vi "SeCrTs-Drive_Read_L.vi"(8 "error in":errorcluster, 9 "Message Queue":refnum<queue>, 11 "Data FIFO Ref":T1) -> (0 "error out":errorcluster)   [LabVIEW 2022 SP3]
uses:
  RT Controls/SeCrTs-Data FIFO.ctl
  RT Support/SeCrTs-RT_Global_R.vi
panel:
  in  "TCP_Port_Bottom":u16=3000
  in  "TCP_Port_Top":u16=2000
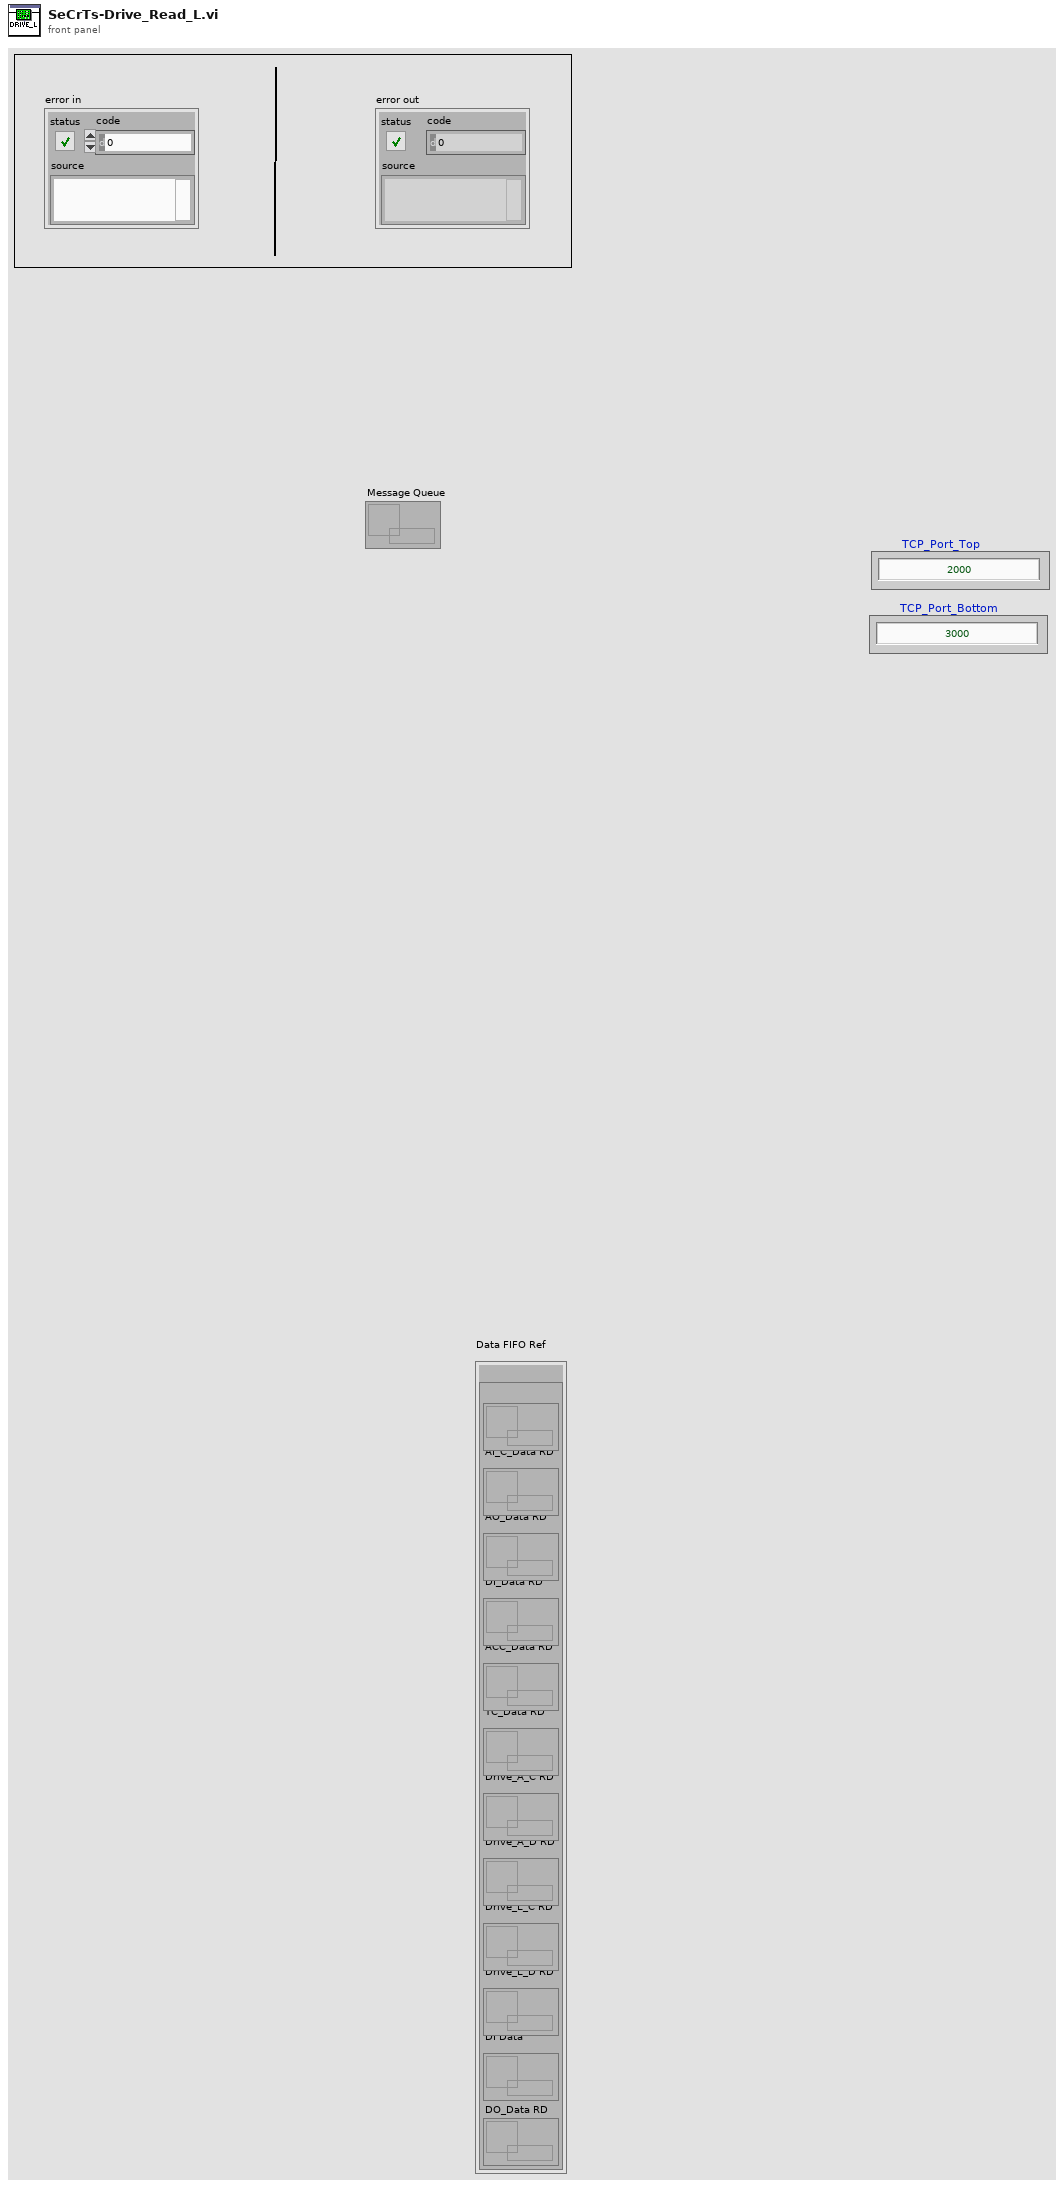
[diagram p1: front panel]
types:
  T1 = typedef "SeCrTs-Data FIFO.ctl" = cluster{"RD":cluster{"AI_V_Data RD":refnum<queue>, "AI_C_Data RD":refnum<queue>, "AO_Data RD":refnum<queue>, "DI_Data RD":refnum<queue>, "ACC_Data RD":refnum<queue>, "TC_Data RD":refnum<queue>, "Drive_A_C RD":refnum<queue>, "Drive_A_D RD":refnum<queue>, "Drive_L_C RD":refnum<queue>, "Drive_L_D RD":refnum<queue>, "DI Data":refnum<queue>, "DO_Data RD":refnum<queue>}}
  T2 = enum16{"AI C", "AI V", "AO", "DI", "DO", "TC", "ACC", "DR L", "DR A"}
  T3 = enum16{"Init", "Read 'All'", "Read 'n'", "Read '1'", "Write '1'", "Write 'n'", "Write 'All'"}
  T4 = cluster{"Start DAQ":bool, "Stop DAQ":bool, "RT Stop":bool, "RT Exit":bool, "Start Seq":bool}
  T5 = cluster{"En_Drive_A":bool, "En_Drive_L":bool, "Exit_Drive_A":bool, "Exit_Drive_L":bool}
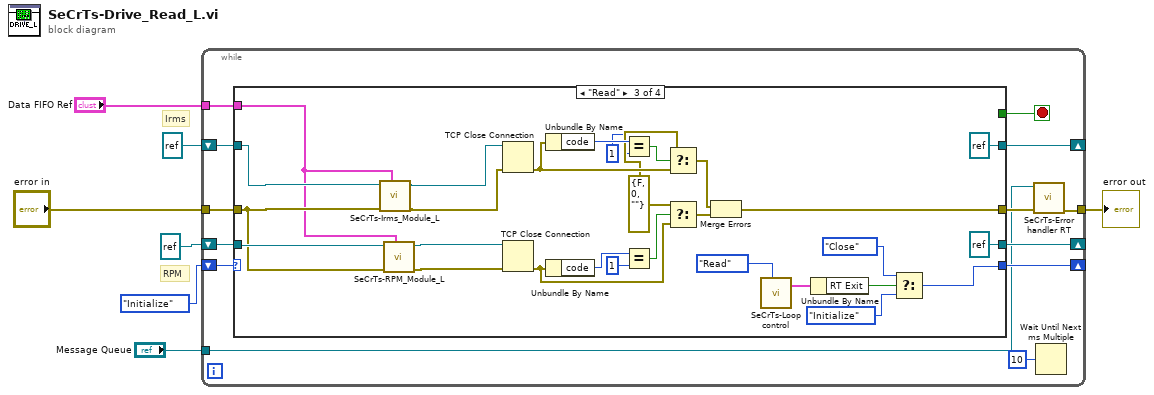
[diagram p0: block diagram]
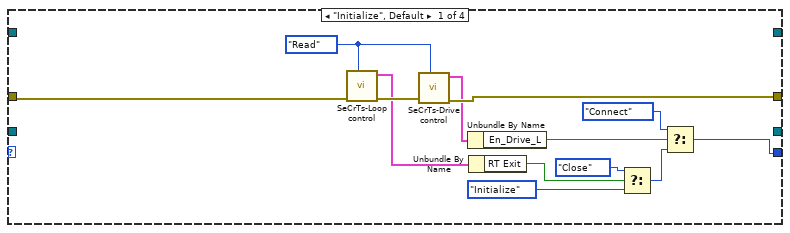
[diagram p2: hidden frame]
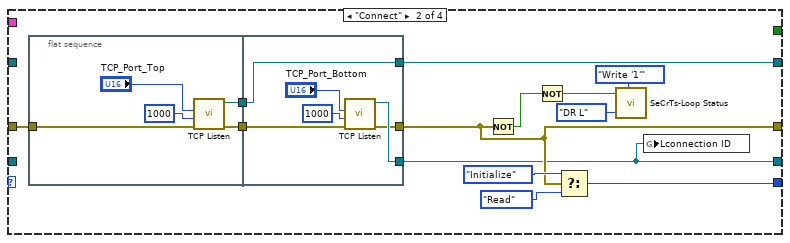
[diagram p3: hidden frame]
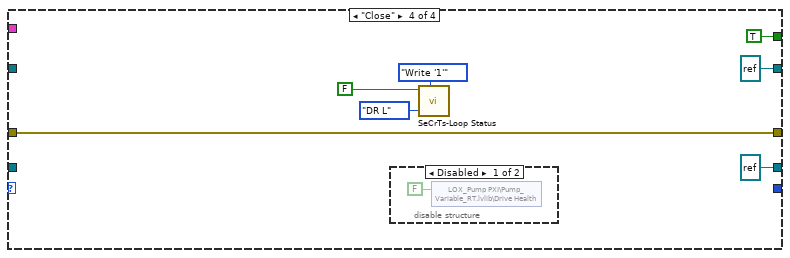
[diagram p4: hidden frame]
diagram:
  # "RPM"
  # "Irms"
  n1 = while {
    shift-right: [w19] -> _
    shift-left: enum16{"Initialize", "Connect", "Read", "Close"}."Initialize" -> [w20]
    tunnel: "error in" -> [w18]
    tunnel: [w10] -> w5
    shift-right: [w17] -> _
    shift-left: refnum<k5> refnum ("connection ID") -> [w15]
    shift-right: [w16] -> _
    shift-left: refnum<k5> refnum ("connection ID") -> [w14]
    tunnel: "Data FIFO Ref" -> [w12]
    tunnel: "Message Queue" -> [w9]
    stop <- w13 stop-if-true
    n2 = case shown="\"Read\"" w20 {
      tunnel: [w33 w40 w83 _] -> w19
      tunnel: w18 -> [w28 w44 w60 w89]
      tunnel: [w26 w39 w71 w89] -> w11
      tunnel: [_ w43 refnum<k5> refnum ("TCP Network Connection out") refnum<k5> refnum ("TCP Network Connection out")] -> w17
      tunnel: [_ w38 refnum<k5> refnum ("TCP Network Connection out") refnum<k5> refnum ("TCP Network Connection out")] -> w16
      tunnel: w15 -> [_ _ w65 _]
      tunnel: w14 -> [_ _ w61 _]
      tunnel: [_ _ _ TRUE] -> w13
      tunnel: w12 -> [_ _ w58 _]
      frame "Initialize", Default {
        w25 = enum16{"Init", "Write", "Read"}."Read" ("Action")
        n3 = call "SeCrTs-Loop control.vi"("Action"=w25, "error in (no error)"=w28) -> ("error Out"=w27:errorcluster, "Loop Control out"=w24:T4)  [unwired: 8 in]
        n4 = call "SeCrTs-Drive control.vi"("Action"=w25, "error in"=w27) -> ("error Out"=w26:errorcluster, "Loop Control Out"=w22:T5)  [unwired: 8 in]
        n5 = Unbundle By Name(w22) -> ("En_Drive_L"=w21:bool)
        n6 = Unbundle By Name(w24) -> ("RT Exit"=w23:bool)
        n7 = Select(t=enum16{"Initialize", "Connect", "Read", "Close"}."Close", s=w23, f=enum16{"Initialize", "Connect", "Read", "Close"}."Initialize") -> (s? t:f=w29:enum16{"Initialize", "Connect", "Read", "Close"})
        n8 = Select(t=enum16{"Initialize", "Connect", "Read", "Close"}."Connect", s=w21, f=w29) -> (s? t:f=w33:enum16{"Initialize", "Connect", "Read", "Close"})
      }
      frame "Connect" {
        n9 = flat-sequence {
          tunnel: w44 -> [w49]
          tunnel: [w48] -> w46
          tunnel: [w47] -> w45
          tunnel: [w57] -> w38
          tunnel: w46 -> [w53]
          tunnel: w45 -> [w56]
          tunnel: [w56] -> w43
          tunnel: [w52] -> w39
          frame #0 {
            n10 = call <vilib>:"TCP Listen.vi"("error in (no error)"=w49, "timeout ms (wait forever: -1)"=1000, "port"="TCP_Port_Top") -> ("error out"=w48:errorcluster, "connection ID"=w47:refnum<k5>)  [unwired: 4 in, 3 out]
          }
          frame #1 {
            n11 = call <vilib>:"TCP Listen.vi"("error in (no error)"=w53, "timeout ms (wait forever: -1)"=1000, "port"="TCP_Port_Bottom") -> ("error out"=w52:errorcluster, "connection ID"=w57:refnum<k5>)  [unwired: 4 in, 3 out]
          }
        }
        n12 = Not(x=w39) -> (.not. x?=w34:bool)
        n13 = Not(x=w34) -> (.not. x?=w36:bool)
        n14 = Select(t=enum16{"Initialize", "Connect", "Read", "Close"}."Initialize", s=w39, f=enum16{"Initialize", "Connect", "Read", "Close"}."Read") -> (s? t:f=w40:enum16{"Initialize", "Connect", "Read", "Close"})
        n15 = call "SeCrTs-Loop Status.vi"("Option"=T3."Write '1'", "Status"=w36, "Loop"=T2."DR L") -> ()  [unwired: 6 in, 3 out]
        n16 = global write "SeCrTs-RT_Global_R.vi" "Lconnection ID"(w38) -> ()
      }
      frame "Read" {
        w74 = errorcluster {"status"=FALSE, "code"=0, "source"=""} ("error constant")
        n17 = call "SeCrTs-Irms_Module_L.vi"("Data FIFO Ref"=w58, "error in"=w60, "TCP Network Connection in"=w65) -> ("error out"=w64:errorcluster, "TCP Network Connection out"=w66:refnum<k5>)  [unwired: 7 in]
        n18 = call "SeCrTs-RPM_Module_L.vi"("Data FIFO Ref"=w58, "error in (no error)"=w60, "TCP Network Connection in"=w61) -> ("error out"=w63:errorcluster, "TCP Network Connection out"=w62:refnum<k5>)  [unwired: 7 in]
        n19 = TCP Close Connection(connection ID=w66, error in (no error)=w64) -> (error out=w78:errorcluster)  [unwired: 1 in, 1 out]
        n20 = TCP Close Connection(connection ID=w62, error in (no error)=w63) -> (error out=w77:errorcluster)  [unwired: 1 in, 1 out]
        n21 = Unbundle By Name(w78) -> ("code"=w82:i32)
        n22 = Unbundle By Name(w77) -> ("code"=w81:i32)
        n23 = Equal?(x=w82, y=1) -> (x = y?=w79:bool)
        n24 = Equal?(x=w81, y=1) -> (x = y?=w80:bool)
        n25 = Select(t=w74, s=w79, f=w78) -> (s? t:f=w76:errorcluster)
        n26 = Select(t=w74, s=w80, f=w77) -> (s? t:f=w75:errorcluster)
        n27 = Merge Errors(w76, w75) -> (w71:errorcluster)
        n28 = call "SeCrTs-Loop control.vi"("Action"=enum16{"Init", "Write", "Read"}."Read") -> ("Loop Control out"=w68:T4)  [unwired: 9 in, 1 out]
        n29 = Unbundle By Name(w68) -> ("RT Exit"=w67:bool)
        n30 = Select(t=enum16{"Initialize", "Connect", "Read", "Close"}."Close", s=w67, f=enum16{"Initialize", "Connect", "Read", "Close"}."Initialize") -> (s? t:f=w83:enum16{"Initialize", "Connect", "Read", "Close"})
      }
      frame "Close" {
        n31 = disable-structure shown="Disabled" {
          frame Disabled {
            n32 = shared-variable "LOX_Pump PXI\\Pump_Variable_RT.lvlib\\Drive Health"(FALSE ("Drive Health")) -> ()  [unwired: 1 in, 1 out]
          }
          frame Enabled {
          }
        }
        n33 = call "SeCrTs-Loop Status.vi"("Option"=T3."Write '1'", "Status"=FALSE, "Loop"=T2."DR L") -> ()  [unwired: 6 in, 3 out]
      }
    }
    n34 = call "SeCrTs-Error handler RT.vi"("error in"=w11, "Message Queue"=w9) -> ("error out"=w10:errorcluster)  [unwired: 8 in, 1 out]
    n35 = Wait Until Next ms Multiple(millisecond multiple=u32 10) -> ()  [unwired: 1 out]
  }
  "error out" <- w5
